vi "Wait.vi"() -> ()   [LabVIEW 2018]
panel:
  out "숫자형 3":i32
  out "숫자형 2":i32
  out "숫자형":i32
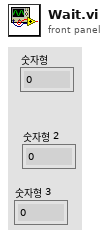
[diagram p1: front panel]
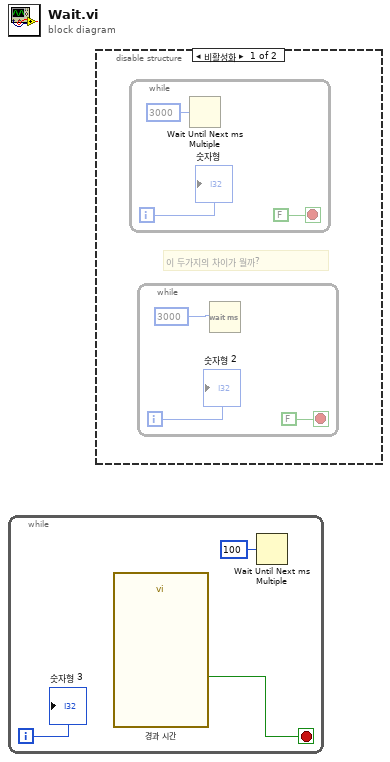
[diagram p0: block diagram]
diagram:
  n1 = while {
    i -> [w1]
    stop <- w2 stop-if-true
    n2 = call "경과 시간"() -> ("Time has Elapsed"=w2:bool)  [unwired: 12 in, 7 out]
    n3 = Wait Until Next ms Multiple(millisecond multiple=u32 100 ("ms 배수")) -> ()  [unwired: 1 out]
    "숫자형 3" <- w1
  }
  n4 = disable-structure shown="비활성화" {
    frame Disabled {
      # "이 두가지의 차이가 뭘까?"
      n5 = while {
        i -> [w7]
        stop <- FALSE stop-if-true
        n6 = Wait Until Next ms Multiple(millisecond multiple=u32 3000 ("ms 배수")) -> ()  [unwired: 1 out]
        "숫자형" <- w7
      }
      n7 = while {
        i -> [w5]
        stop <- FALSE stop-if-true
        n8 = Wait (ms)(milliseconds to wait=u32 3000 ("ms 배수")) -> ()  [unwired: 1 out]
        "숫자형 2" <- w5
      }
    }
    frame Enabled {
    }
  }
